vi "Sequence-Started.vi"(8 "error in (no error)":errorcluster, 11 "MCListbox Refnum":refnum<vi>) -> (0 "error out":errorcluster, 3 "MCListbox Refnum(dup)":refnum<vi>)   [LabVIEW 2020, in "CSMScript-Engine(Lite).lvlib"]
uses:
  CSMScript-Engine(Lite).lvlib
panel:
  # "Connector Pane"
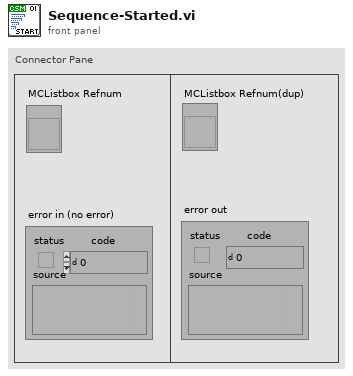
[diagram p1: front panel]
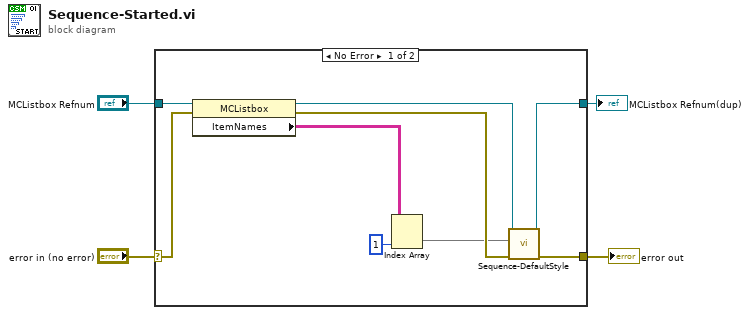
[diagram p0: block diagram]
diagram:
  n1 = case shown="No Error" "error in (no error)" {
    selector: "error in (no error)" -> [w12 w15]
    tunnel: [w9 w15] -> w4
    tunnel: "MCListbox Refnum" -> [w13 w14]
    tunnel: [w8 w14] -> w1
    frame No Error {
      n2 = property class="MCListbox"(reference=w13, error in=w12) -> (reference out=w11:refnum<vi>, error out=w10:errorcluster, "ItemNames"=w7:string[][])
      n3 = Index Array(array=w7, index (col)=1 ("disabled index (col)")) -> (element=w5:string[])  [unwired: 1 in]
      n4 = call "Sequence-DefaultStyle.vi"("error in (no error)"=w10, "Test Steps"=w5, "MCListbox Refnum"=w11) -> ("error out"=w9:errorcluster, "MCListbox Refnum(dup)"=w8:refnum<vi>)  [unwired: 7 in]
    }
    frame Error {
    }
  }
  "error out" <- w4
  "MCListbox Refnum(dup)" <- w1
